vi "Authenticate.vi"(8 "error in (no error)":errorcluster, 10 "Authentication Info":T1, 11 "Scope Needed?":T2) -> (0 "error out":errorcluster, 2 "Timeout":dbl, 3 "Access Token":string)   [LabVIEW 2016]
uses:
  scope_needed.ctl
  OAuth/OAuth.lvclass
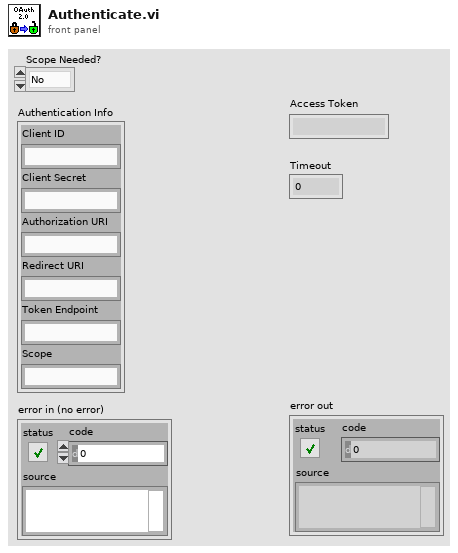
[diagram p1: front panel]
types:
  T1 = cluster{"Client ID":string, "Client Secret":string, "Authorization URI":string, "Redirect URI":string, "Token Endpoint":string, "Scope":string}
  T2 = typedef "scope_needed.ctl" = enum16{"No", "Yes"}
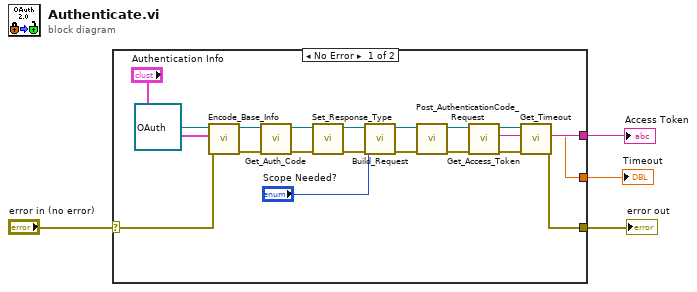
[diagram p0: block diagram]
diagram:
  n1 = case shown="No Error" "error in (no error)" {
    selector: "error in (no error)" -> [w23 w24]
    tunnel: [w11 w24] -> w3
    tunnel: [w10 _] -> w2
    tunnel: [w9 _] -> w1
    frame No Error {
      n2 = call "Encode_Base_Info.vi"("error in (no error)"=w23, "Authentication Info"="Authentication Info", "OAuth in"=refnum<class "OAuth.lvclass"> refnum ("OAuth.lvclass")) -> ("error out"=w18:errorcluster, "OAuth out"=w19:refnum<class "OAuth.lvclass">)  [unwired: 7 in]
      n3 = call-dynamic "Get_Auth_Code.vi"("error in (no error)"=w18, "OAuth in"=w19) -> ("error out"=w7:errorcluster, "OAuth out"=w8:refnum<class "OAuth.lvclass">)  [unwired: 8 in]
      n4 = call "Set_Response_Type.vi"("error in (no error)"=w7, "OAuth in"=w8) -> ("error out"=w6:errorcluster, "OAuth out"=w5:refnum<class "OAuth.lvclass">)  [unwired: 8 in]
      n5 = call-dynamic "Build_Request.vi"("error in (no error)"=w6, "Application"="Scope Needed?", "OAuth in"=w5) -> ("error out"=w16:errorcluster, "OAuth out"=w17:refnum<class "OAuth.lvclass">)  [unwired: 7 in]
      n6 = call-dynamic "Post_AuthenticationCode_Request.vi"("error in (no error)"=w16, "OAuth in"=w17) -> ("error out"=w15:errorcluster, "OAuth out"=w13:refnum<class "OAuth.lvclass">)  [unwired: 8 in]
      n7 = call-dynamic "Get_Access_Token.vi"("error in (no error)"=w15, "OAuth in"=w13) -> ("error out"=w14:errorcluster, "Access Token"=w10:string, "OAuth out"=w12:refnum<class "OAuth.lvclass">)  [unwired: 7 in]
      n8 = call-dynamic "Get_Timeout.vi"("error in (no error)"=w14, "OAuth in"=w12) -> ("error out"=w11:errorcluster, "Timeout"=w9:dbl)  [unwired: 7 in, 1 out]
    }
    frame Error {
    }
  }
  "error out" <- w3
  "Access Token" <- w2
  "Timeout" <- w1
